vi "SetMethodTreeCaption.vi"(9 "MethodsDisabledPerInt":cluster{"Array":bool[]}[](array[cluster]), 10 "MethodsSelectedPerInt":cluster{"Array":bool[]}[](array[cluster]), 11 "TreeControl in":refnum<vi>) -> (3 "Methods will be created":bool)   [LabVIEW 2020, in "InterfaceLibrary.lvlib"]
uses:
  <resource>/Framework/Providers/Open_GDS/ClassProviders/Common/InterfaceLibrary/InterfaceLibrary.lvlib
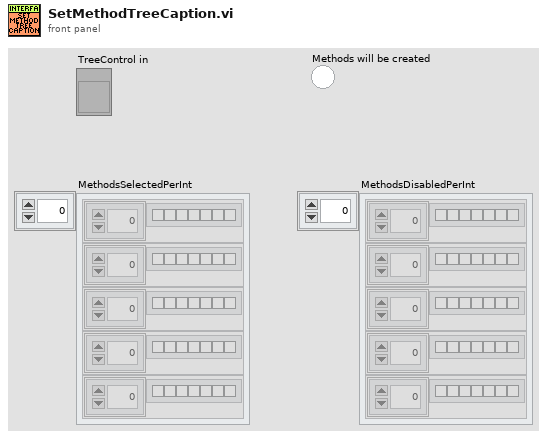
[diagram p1: front panel]
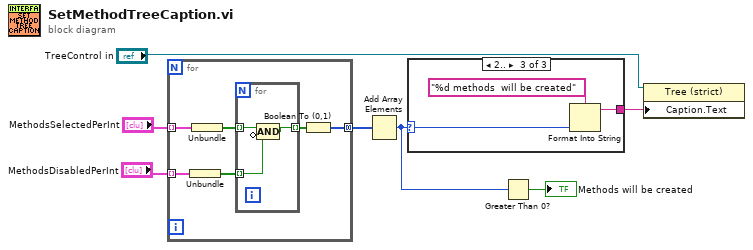
[diagram p0: block diagram]
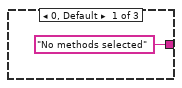
[diagram p2: hidden frame]
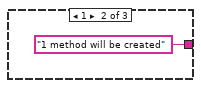
[diagram p3: hidden frame]
diagram:
  n1 = for {
    tunnel: "MethodsSelectedPerInt" -> [w13] mode=indexing
    tunnel: [w12] -> w6 mode=concatenating
    tunnel: "MethodsDisabledPerInt" -> [w11] mode=indexing
    n2 = Unbundle(w11) -> ("Array"=w9:bool[])
    n3 = Unbundle(w13) -> ("Array"=w10:bool[])
    n4 = for {
      tunnel: w10 -> [w16] mode=indexing
      tunnel: w9 -> [w15] mode=indexing
      tunnel: [w14] -> w8 mode=indexing
      n5 = Compound Arithmetic op=AND(w16, invert w15) -> (w14:bool)
    }
    n6 = Boolean To (0,1)(Boolean=w8) -> (0, 1=w12:i16[])
  }
  n7 = Add Array Elements(numeric array=w6) -> (sum=w2:i16)
  n8 = case shown="2.." w2 {
    selector: w2 -> [_ _ w19]
    tunnel: ["No methods selected" ("regular expression") "1 method will be created" ("regular expression") w20] -> w5
    frame 0, Default {
    }
    frame 1 {
    }
    frame 2.. {
      n9 = Format Into String(format string="%d methods  will be created" ("regular expression"), w19) -> (resulting string=w20:string)  [unwired: 2 in, 1 out]
    }
  }
  n10 = Greater Than 0?(x=w2) -> (x > 0?=→"Methods will be created":bool)
  n11 = property on="Property Node" class="Tree (strict)"(reference="TreeControl in", "Caption.Text"=w5) -> ()  [unwired: 1 in, 2 out]
